vi "Gcode simulator.vi"() -> ()   [LabVIEW 2020]
panel:
  out "XY Graph":cluster{"X":dbl, "Y":dbl}[](graph)
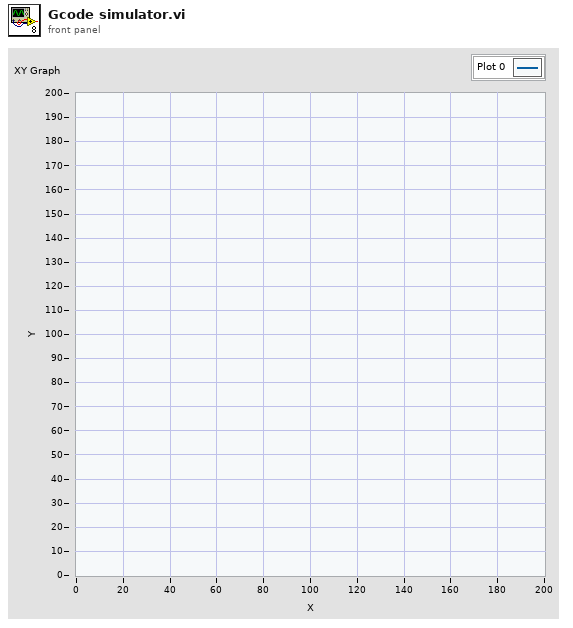
[diagram p1: front panel]
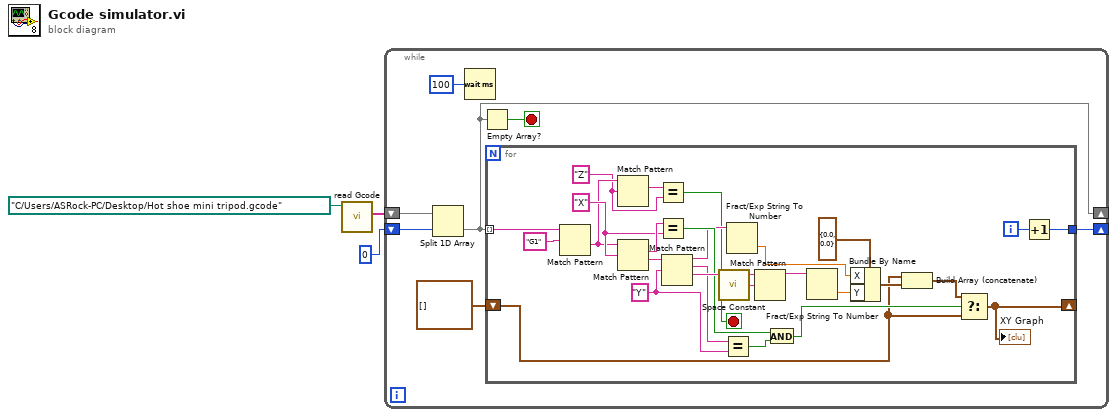
[diagram p0: block diagram]
diagram:
  n1 = call "read Gcode.vi"("Gcode path (use dialog)"=path "C:/Users/ASRock-PC/Desktop/Hot shoe mini tripod.gcode") -> ("Gcode Array"=w3:string[])  [unwired: 8 in, 2 out]
  n2 = while {
    shift-right: [w10] -> _
    shift-left: 0 -> [w8]
    shift-right: [w5] -> _
    shift-left: w3 -> [w9]
    stop <- w7 stop-if-true
    n3 = Split 1D Array(array=w9, index=w8) -> (second subarray=w5:string[])  [unwired: 1 out]
    n4 = Wait (ms)(milliseconds to wait=u32 100) -> ()  [unwired: 1 out]
    n5 = Empty Array?(array=w5) -> (empty?=w7:bool)
    n6 = for {
      tunnel: w5 -> [w37] mode=indexing
      tunnel: [w16] -> w10
      shift-right: [w11] -> _
      shift-left: cluster{"X":dbl, "Y":dbl}[] [] ("XY Graph 2") -> [w12]
      i -> [w17]
      stop <- w18 stop-if-true
      w19 = "Z" ("regular expression")
      w29 = "Y" ("regular expression")
      w31 = "X" ("regular expression")
      n7 = Match Pattern(string=w37, regular expression="G1") -> (after substring=w21:string)  [unwired: 1 in, 3 out]
      n8 = Match Pattern(string=w21, regular expression=w19) -> (match substring=w20:string)  [unwired: 1 in, 3 out]
      n9 = Match Pattern(string=w21, regular expression=w31) -> (match substring=w32:string, after substring=w35:string)  [unwired: 1 in, 2 out]
      n10 = Equal?(x=w20, y=w19) -> (x = y?=w18:bool)
      n11 = Equal?(x=w32, y=w31) -> (x = y?=w28:bool)
      n12 = Match Pattern(string=w35, regular expression=w29) -> (before substring=w26:string, match substring=w30:string, after substring=w34:string)  [unwired: 1 in, 1 out]
      n13 = call <vilib>:"Space Constant.vi"() -> ("String"=w33:string)
      n14 = Equal?(x=w30, y=w29) -> (x = y?=w27:bool)
      n15 = Fract/Exp String To Number(string=w26) -> (number=w23:dbl)  [unwired: 3 in, 1 out]
      n16 = Match Pattern(string=w34, regular expression=w33) -> (before substring=w25:string)  [unwired: 1 in, 3 out]
      n17 = And(x=w28, y=w27) -> (x .and. y?=w15:bool)
      n18 = Fract/Exp String To Number(string=w25) -> (number=w22:dbl)  [unwired: 3 in, 1 out]
      n19 = Bundle By Name(cluster=cluster{"X":dbl, "Y":dbl} {"X"=0.0, "Y"=0.0} ("XY Graph"), "X"=w23, "Y"=w22) -> (w13:cluster{"X":dbl, "Y":dbl})
      n20 = Build Array (concatenate)(w12, w13) -> (w14:cluster{"X":dbl, "Y":dbl}[])
      n21 = Select(t=w14, s=w15, f=w12) -> (s? t:f=w11:cluster{"X":dbl, "Y":dbl}[])
      "XY Graph" <- w11
      n22 = Increment(x=w17) -> (x+1=w16:i32)
    }
  }
